vi "Centripetal Acc Correction.vi"(9 "Time Delta":dbl, 10 "Max Centripetal Acc":dbl, 11 "Motion Cluster":T1(array[cluster])) -> (3 "Corrected Motion Cluster":T1(array[cluster]))   [LabVIEW 2016]
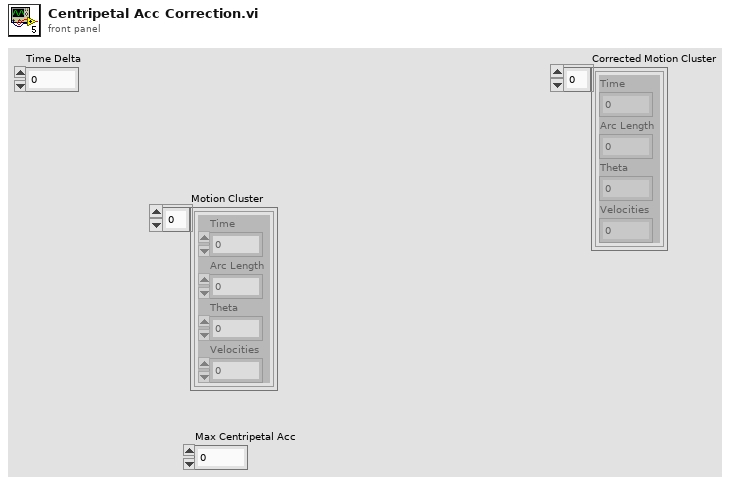
[diagram p1: front panel]
types:
  T1 = cluster{"Time":dbl, "Arc Length":dbl, "Theta":dbl, "Velocities":dbl}[]
  T2 = cluster{"Time":dbl, "Arc Length":dbl, "Theta":dbl, "Velocities":dbl}
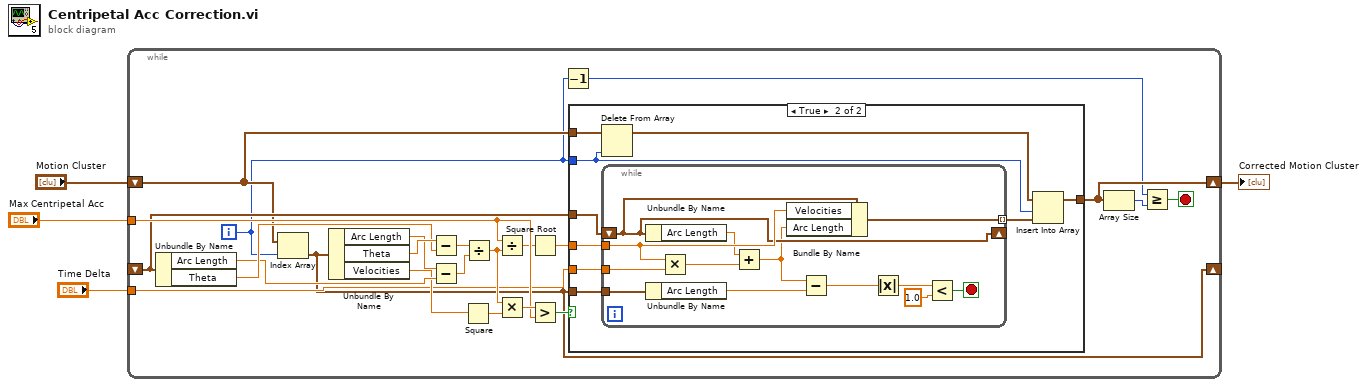
[diagram p0: block diagram]
diagram:
  n1 = while {
    shift-right: [w11] -> _
    shift-left: _ -> [w12]
    tunnel: "Max Centripetal Acc" -> [w17]
    tunnel: "Time Delta" -> [w13]
    shift-right: [w8] -> w1
    shift-left: "Motion Cluster" -> [w10]
    i -> [w9]
    stop <- w6 stop-if-true
    n2 = Unbundle By Name(w12) -> ("Arc Length"=w24:dbl, "Theta"=w26:dbl)
    n3 = Index Array(array=w10, index=w9) -> (element=w11:T2)
    n4 = Unbundle By Name(w11) -> ("Arc Length"=w25:dbl, "Theta"=w27:dbl, "Velocities"=w21:dbl)
    n5 = Subtract(x=w27, y=w26) -> (x-y=w23:dbl)
    n6 = Subtract(x=w25, y=w24) -> (x-y=w22:dbl)
    n7 = Square(x=w21) -> (x^2=w20:dbl)
    n8 = Divide(x=w23, y=w22) -> (x/y=w18:dbl)
    n9 = Divide(x=w17, y=w18) -> (x/y=w16:dbl)
    n10 = Multiply(x=w18, y=w20) -> (x*y=w19:dbl)
    n11 = Square Root(x=w16) -> (sqrt(x)=w14:dbl)
    n12 = Greater?(x=w19, y=w17) -> (0:w15:bool)
    n13 = Decrement(x=w9) -> (x-1=w5:i32)
    n14 = case shown="True" w15 {
      tunnel: w14 -> [_ w37]
      tunnel: w13 -> [_ w36]
      tunnel: w12 -> [_ w35]
      tunnel: w11 -> [_ w34]
      tunnel: w10 -> [w28 w32]
      tunnel: w9 -> [_ w30]
      tunnel: [w28 w29] -> w8
      frame False {
      }
      frame True {
        n15 = Delete From Array(array=w32, index=w30) -> (array with subset deleted=w31:T1)  [unwired: 1 in, 1 out]
        n16 = while {
          tunnel: w37 -> [w50]
          tunnel: w36 -> [w49]
          shift-right: [w46] -> _
          shift-left: w35 -> [w46]
          tunnel: w34 -> [w44]
          tunnel: [w38] -> w33 mode=indexing
          stop <- w39 stop-if-true
          n17 = Unbundle By Name(w46) -> ("Arc Length"=w47:dbl)
          n18 = Unbundle By Name(w44) -> ("Arc Length"=w43:dbl)
          n19 = Multiply(x=w50, y=w49) -> (x*y=w48:dbl)
          n20 = Add(x=w47, y=w48) -> (x+y=w45:dbl)
          n21 = Bundle By Name(cluster=w46, "Velocities"=w50, "Arc Length"=w45) -> (w38:T2)
          n22 = Subtract(x=w45, y=w43) -> (x-y=w42:dbl)
          n23 = Absolute Value(x=w42) -> (abs(x)=w41:dbl)
          n24 = Less?(x=w41, y=1.0) -> (x < y?=w39:bool)
        }
        n25 = Insert Into Array(array=w31, index=w30, new element=w33) -> (w29:T1)
      }
    }
    n26 = Array Size(array=w8) -> (size(s)=w7:i32)
    n27 = Greater Or Equal?(x=w5, y=w7) -> (x >= y?=w6:bool)
  }
  "Corrected Motion Cluster" <- w1
